vi "Wire Release Sessions.vi"(0 "logiv vi ref":refnum<vi>, 5 "sub vis ref":refnum<vi>[](array[refnum]), 11 "error in":errorcluster) -> (15 "error out":errorcluster)   [LabVIEW 2021, in "Converter.lvlib"]
uses:
  Converter.lvlib
  Converter Reusables/Converter Reusables.lvlib
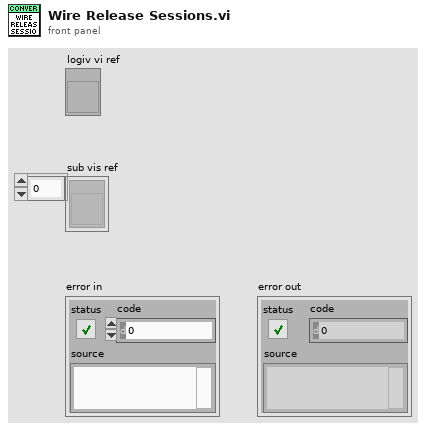
[diagram p1: front panel]
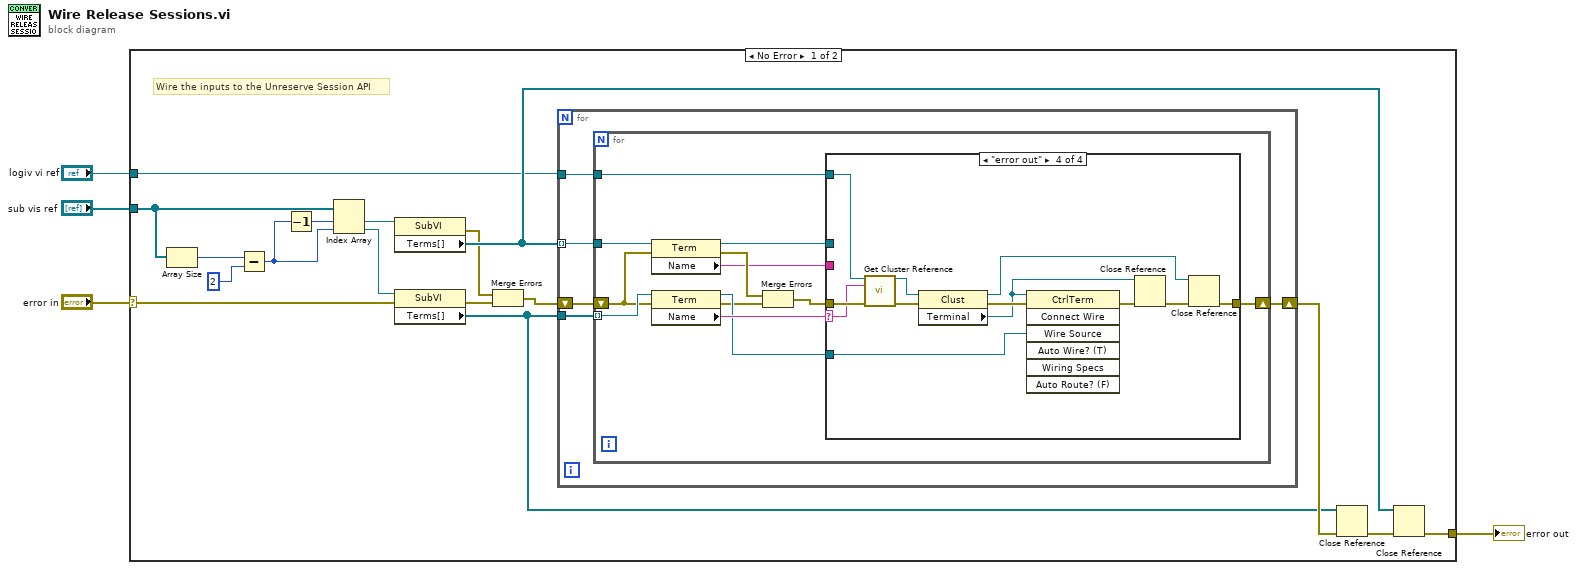
[diagram p0: block diagram]
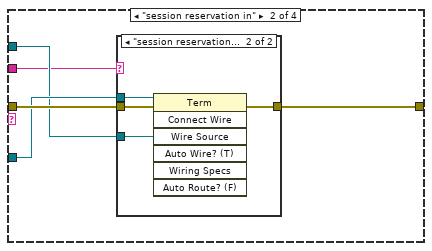
[diagram p3: hidden frame]
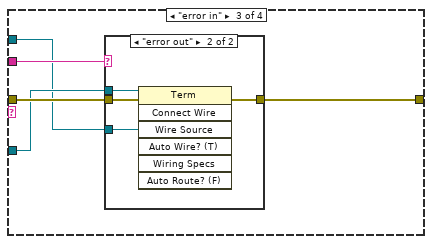
[diagram p5: hidden frame]
diagram:
  n1 = case shown="No Error" "error in" {
    selector: "error in" -> [w21 w72]
    tunnel: [w5 w72] -> w4
    tunnel: "logiv vi ref" -> [w15 _]
    tunnel: "sub vis ref" -> [w11 _]
    frame No Error {
      # "Wire the inputs to the Unreserve Session API"
      n2 = Array Size(array=w11) -> (size(s)=w10:i32)
      n3 = Subtract(x=w10, y=2) -> (x-y=w7:i32)
      n4 = Decrement(x=w7) -> (x-1=w8:i32)
      n5 = Index Array(array=w11, index #1=w8, index #2=w7) -> (element #1=w16:refnum<vi>, element #2=w12:refnum<vi>)
      n6 = property class="SubVI"(reference=w16) -> (error out=w14:errorcluster, "Terms[]"=w17:refnum<vi>[])  [unwired: 1 in, 1 out]
      n7 = property class="SubVI"(reference=w12, error in=w21) -> (error out=w20:errorcluster, "Terms[]"=w6:refnum<vi>[])  [unwired: 1 out]
      n8 = Merge Errors(w14, w20) -> (w13:errorcluster)
      n9 = for {
        tunnel: w17 -> [w25] mode=indexing
        tunnel: w6 -> [w26]
        tunnel: w15 -> [w23]
        shift-right: [w22] -> w19
        shift-left: w13 -> [w24]
        n10 = for {
          tunnel: w26 -> [w29] mode=indexing
          tunnel: w25 -> [w38]
          tunnel: w23 -> [w32]
          shift-right: [w33] -> w22
          shift-left: w24 -> [w28]
          n11 = property class="Term"(reference=w38, error in=w28) -> (reference out=w34:refnum<vi>, error out=w30:errorcluster, "Name"=w27:string)
          n12 = property class="Term"(reference=w29, error in=w28) -> (reference out=w36:refnum<vi>, error out=w35:errorcluster, "Name"=w37:string)
          n13 = Merge Errors(w30, w35) -> (w31:errorcluster)
          n14 = case shown="\"error out\"" w37 {
            selector: w37 -> [_ _ _ w61]
            tunnel: w27 -> [_ w40 w54 _]
            tunnel: w36 -> [_ w43 w52 w64]
            tunnel: w31 -> [w39 w44 w53 w70]
            tunnel: [w39 w41 w51 w65] -> w33
            tunnel: w34 -> [_ w42 w50 _]
            tunnel: w32 -> [_ _ _ w71]
            frame Default {
            }
            frame "session reservation in" {
              n15 = case shown="\"session reservation out\"" w40 {
                tunnel: w44 -> [w45 w49]
                tunnel: w43 -> [_ w48]
                tunnel: w42 -> [_ w46]
                tunnel: [w45 w47] -> w41
                frame Default {
                }
                frame "session reservation out" {
                  n16 = invoke class="Term" method="Connect Wire"(reference=w48, error in=w49, "Wire Source"=w46) -> (error out=w47:errorcluster)  [unwired: 4 in, 6 out]
                }
              }
            }
            frame "error in" {
              n17 = case shown="\"error out\"" w54 {
                tunnel: w53 -> [w55 w59]
                tunnel: w52 -> [_ w58]
                tunnel: [w55 w57] -> w51
                tunnel: w50 -> [_ w56]
                frame Default {
                }
                frame "error out" {
                  n18 = invoke class="Term" method="Connect Wire"(reference=w58, error in=w59, "Wire Source"=w56) -> (error out=w57:errorcluster)  [unwired: 4 in, 6 out]
                }
              }
            }
            frame "error out" {
              n19 = call "Get Cluster Reference.vi"("vi in"=w71, "name/order"=w61, "error in"=w70) -> ("cluster out"=w60:refnum<vi>, "error out"=w69:errorcluster)  [unwired: 11 in]
              n20 = property class="Clust"(reference=w60, error in=w69) -> (reference out=w63:refnum<vi>, error out=w68:errorcluster, "Terminal"=w62:refnum<vi>)
              n21 = invoke class="CtrlTerm" method="Connect Wire"(reference=w62, error in=w68, "Wire Source"=w64) -> (error out=w67:errorcluster)  [unwired: 4 in, 6 out]
              n22 = Close Reference(reference=w62, error in (no error)=w67) -> (error out=w66:errorcluster)
              n23 = Close Reference(reference=w63, error in (no error)=w66) -> (error out=w65:errorcluster)
            }
          }
        }
      }
      n24 = Close Reference(reference=w6, error in (no error)=w19) -> (error out=w18:errorcluster)
      n25 = Close Reference(reference=w17, error in (no error)=w18) -> (error out=w5:errorcluster)
    }
    frame Error {
    }
  }
  "error out" <- w4
